vi "Tosca-Enumerate Rigs.vi"() -> (8 "Rigs":string[](array[string]))   [LabVIEW 2020]
uses:
  <vilib>/Utility/sysdir.llb/System Directory Type.ctl
  <vilib>/regexp/Match Regular Expression.xnode
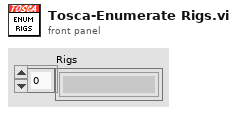
[diagram p1: front panel]
types:
  T1 = typedef "System Directory Type.ctl" = i32
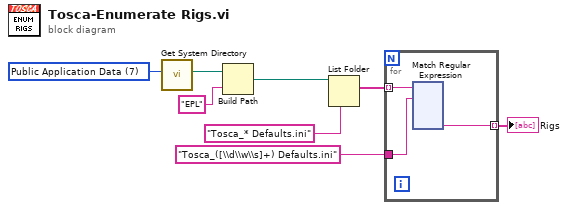
[diagram p0: block diagram]
diagram:
  w7 = T1 7 items=["User Home", "User Desktop", "User Documents", "User Application Data", "User Preferences", "User Temporary", "Public Documents", "Public Application Data", "Public Preferences", "System Core Libraries", "System Installed Libraries", "Application Files", "Boot Volume Root"] ("system directory type")
  n1 = call <vilib>:"Get System Directory.vi"("system directory type"=w7) -> ("system directory"=w8:path)  [unwired: 10 in]
  n2 = Build Path(base path=w8, name or relative path="EPL") -> (appended path=w5:path)
  n3 = List Folder(path=w5, pattern="Tosca_* Defaults.ini") -> (filenames=w3:string[])  [unwired: 2 in, 3 out]
  n4 = for {
    tunnel: w3 -> [w11] mode=indexing
    tunnel: "Tosca_([\\d\\w\\s]+) Defaults.ini" ("pattern") -> [w10]
    tunnel: [w9] -> w1 mode=indexing
    n5 = xnode "Match Regular Expression"("input string"=w11, "regular expression"=w10) -> ("submatch 1"=w9:string)  [unwired: 4 in, 5 out]
  }
  "Rigs" <- w1
